vi "Ch_names_to_rows.vi"(1 "Channel Names":string[](array[string])) -> (0 "3 Row names":string[][](array[string]))   [LabVIEW 2010]
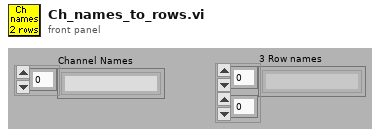
[diagram p1: front panel]
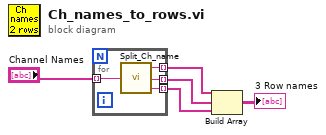
[diagram p0: block diagram]
diagram:
  n1 = for {
    tunnel: "Channel Names" -> [w9] mode=indexing
    tunnel: [w8] -> w1 mode=indexing
    tunnel: [w7] -> w2 mode=indexing
    tunnel: [w6] -> w3 mode=indexing
    n2 = call "Split_Ch_name.vi"("Ch name"=w9) -> ("Top level"=w8:string, "Middle"=w7:string, "Low level"=w6:string)
  }
  n3 = Build Array(w1, w2, w3) -> (→"3 Row names":string[][])
